vi "Send and Receive Message.vi"(6 "timeout (ms) [500]":i32=500, 8 "error in (no error)":errorcluster, 9 "Data":variant, 10 "Command":string, 11 "RemoteControl in":refnum<class "RemoteControl.lvclass">) -> (0 "error out":errorcluster, 1 "Data out":string, 2 "Command out":string, 3 "RemoteControl out":refnum<class "RemoteControl.lvclass">)   [LabVIEW 2019, in "RemoteControl.lvlib" / "RemoteControl.lvclass"]
uses:
  RemoteControl.lvclass
  RemoteControl.lvclass/RemoteControl.ctl
  Typedefs/Message--Cluster.ctl
  09999a43-c557-48ae-b564-ba31de2423f0.vi
  09999a43-c557-48ae-b564-ba31de2423f0.vi/7d2a1554-b401-40ca-9492-c05f0c7b2adc.vi
  09999a43-c557-48ae-b564-ba31de2423f0.vi/449cb8fe-25b7-4578-a4bb-cc8db75334a4.vi
  <vilib>/Utility/Data Type/Get Type Information.vi
  <vilib>/JDP Science/JSONtext/JSON text to Variant.vi
  <vilib>/JDP Science/JSONtext/LVClass Serializer/JSONtext LVClass Serializer.lvclass
panel:
  out "ID":string
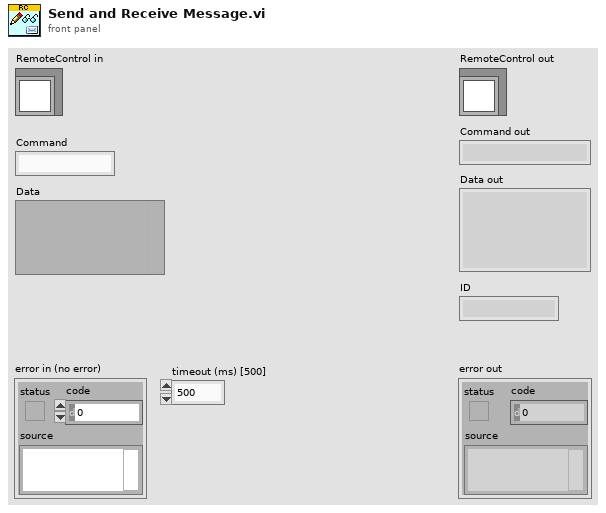
[diagram p1: front panel]
types:
  T1 = typedef "RemoteControl.lvlib/RemoteControl.lvclass/Message--Cluster.ctl" = cluster{"Command":string, "Data":variant, "ID":string, "error":errorcluster}
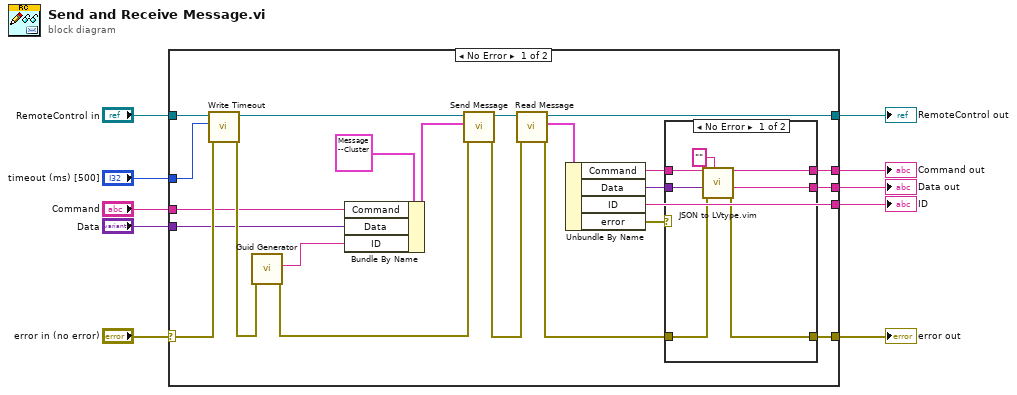
[diagram p0: block diagram]
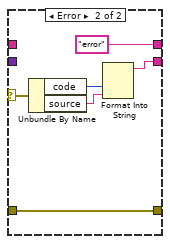
[diagram p2: hidden frame]
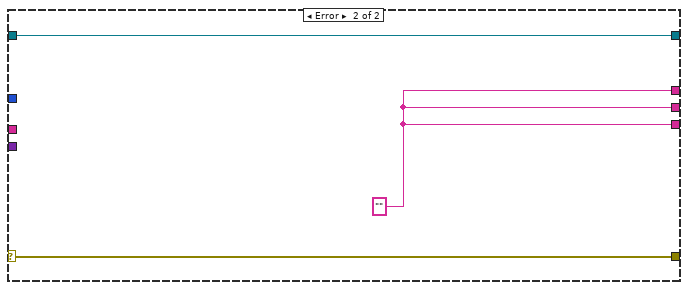
[diagram p3: hidden frame]
diagram:
  n1 = case shown="No Error" "error in (no error)" {
    selector: "error in (no error)" -> [w27 w48]
    tunnel: [w15 w48] -> w10
    tunnel: [w32 w47] -> w8
    tunnel: "RemoteControl in" -> [w29 w47]
    tunnel: "Command" -> [w23 _]
    tunnel: "Data" -> [w21 _]
    tunnel: [w12 w46] -> w5
    tunnel: [w14 w46] -> w1
    tunnel: [w18 w46] -> w4
    tunnel: "timeout (ms) [500]" -> [w30 _]
    frame No Error {
      n2 = call "Write Timeout.vi"("error in (no error)"=w27, "timeout (ms) [500]"=w30, "RemoteControl in"=w29) -> ("error out"=w26:errorcluster, "RemoteControl out"=w28:refnum<class "RemoteControl.lvclass">)  [unwired: 7 in]
      n3 = call <vilib>:"Guid Generator.vi"("error in (no error)"=w26) -> ("error out"=w25:errorcluster, "GUID"=w22:string)  [unwired: 9 in]
      n4 = Bundle By Name(cluster=T1 {"Command"="", "Data"=variant(string ""), "ID"="", "error"={"status"=FALSE, "code"=0, "source"=""}} ("Message"), "Command"=w23, "Data"=w21, "ID"=w22) -> (w20:T1)
      n5 = call-dynamic "Send Message.vi"("error in (no error)"=w25, "Message"=w20, "RemoteControl in"=w28) -> ("error out"=w31:errorcluster, "RemoteControl out"=w33:refnum<class "RemoteControl.lvclass">)  [unwired: 7 in]
      n6 = call-dynamic "Read Message.vi"("error in (no error)"=w31, "RemoteControl in"=w33) -> ("error out"=w16:errorcluster, "Message"=w19:T1, "RemoteControl out"=w32:refnum<class "RemoteControl.lvclass">)  [unwired: 7 in]
      n7 = Unbundle By Name(w19) -> ("Command"=w11:string, "Data"=w17:variant, "ID"=w18:string, "error"=w13:errorcluster)
      n8 = case shown="No Error" w13 {
        selector: w13 -> [_ w45]
        tunnel: w17 -> [w39 _]
        tunnel: w16 -> [w38 w44]
        tunnel: [w37 w44] -> w15
        tunnel: [w36 w40] -> w14
        tunnel: [w34 "error"] -> w12
        tunnel: w11 -> [w34 _]
        frame No Error {
          n9 = call "JSON to LVtype.vim"("type"="", "error in (no error)"=w38, "JSON Data in"=w39) -> ("error out"=w37:errorcluster, "Data out"=w36:string)  [unwired: 7 in]
        }
        frame Error {
          n10 = Unbundle By Name(w45) -> ("code"=w42:i32, "source"=w41:string)
          n11 = Format Into String(w42, w41) -> (resulting string=w40:string)  [unwired: 3 in, 1 out]
        }
      }
    }
    frame Error {
      w46 = "" ("Command")
    }
  }
  "error out" <- w10
  "RemoteControl out" <- w8
  "Command out" <- w5
  "Data out" <- w1
  "ID" <- w4
